vi "Set Button States.vi"(9 "Button States":T1[](array[typedef]), 11 "Button References":refnum<vi>[](array[refnum])) -> ()   [LabVIEW 2018]
doc: "This VI will set the states of the buttons and\nthe enabled, disabled states of the buttons.\n\nThe arrays are assumed to be in the same order"
uses:
  Controls/Button state.ctl
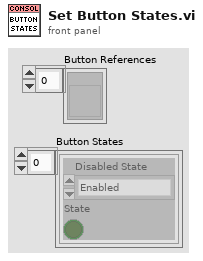
[diagram p1: front panel]
types:
  T1 = typedef "Button state.ctl" = cluster{"Disabled State":enum8{"Enabled", "Disabled", "Disabled and Grayed Out"}, "State":bool}
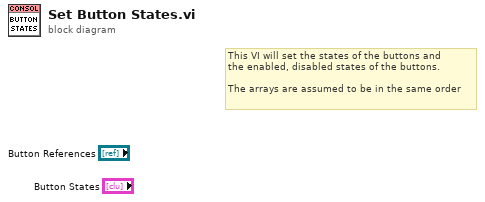
[diagram p0: block diagram]
diagram:
  # "This VI will set the states of the buttons and\nthe enabled, disabled states of the buttons.\n\nThe arrays are assumed to be in the same order"
